vi "Autonomous Turn with Error.vi"(4 "Angle":dbl, 5 "Left Input":dbl, 6 "% Error Margin":dbl, 7 "Right Input":dbl) -> (0 "Left Output":dbl, 1 "Right Output":dbl)   [LabVIEW 2013]
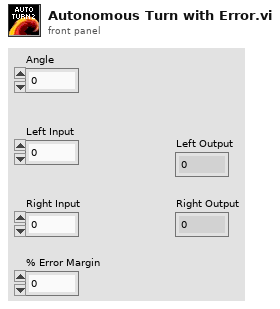
[diagram p1: front panel]
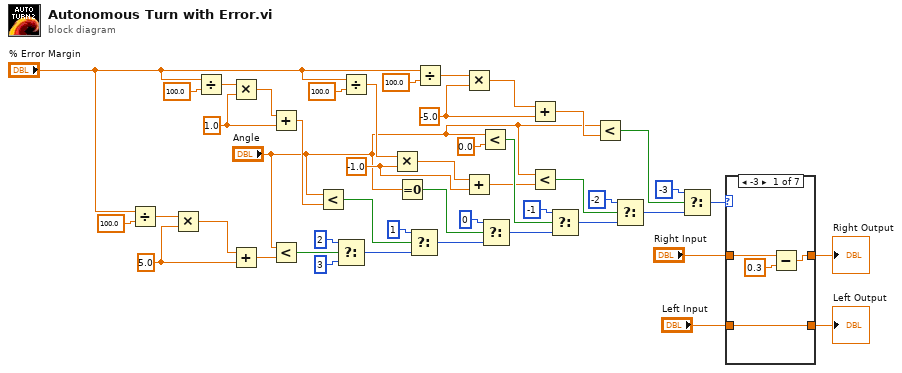
[diagram p0: block diagram]
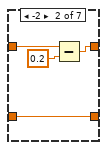
[diagram p2: hidden frame]
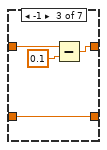
[diagram p3: hidden frame]
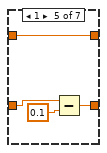
[diagram p5: hidden frame]
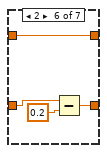
[diagram p6: hidden frame]
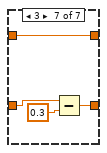
[diagram p7: hidden frame]
diagram:
  w5 = -5.0 ("y")
  w11 = -1.0 ("y")
  w17 = 1.0 ("y")
  w23 = 5.0 ("y")
  n1 = Divide(x="% Error Margin", y=100.0) -> (x/y=w25:dbl)
  n2 = Multiply(x=w25, y=w23) -> (x*y=w24:dbl)
  n3 = Divide(x="% Error Margin", y=100.0) -> (x/y=w19:dbl)
  n4 = Multiply(x=w19, y=w17) -> (x*y=w18:dbl)
  n5 = Add(x=w24, y=w23) -> (x+y=w22:dbl)
  n6 = Add(x=w18, y=w17) -> (x+y=w16:dbl)
  n7 = Less?(x="Angle", y=w22) -> (x < y?=w21:bool)
  n8 = Less?(x="Angle", y=w16) -> (x < y?=w15:bool)
  n9 = Select(t=i8 2, s=w21, f=i8 3) -> (s? t:f=w39:i8)
  n10 = Divide(x="% Error Margin", y=100.0) -> (x/y=w13:dbl)
  n11 = Multiply(x=w13, y=w11) -> (x*y=w12:dbl)
  n12 = Equal To 0?(x="Angle") -> (x = 0?=w35:bool)
  n13 = Select(t=i8 1, s=w15, f=w39) -> (s? t:f=w33:i8)
  n14 = Divide(x="% Error Margin", y=100.0) -> (x/y=w7:dbl)
  n15 = Multiply(x=w7, y=w5) -> (x*y=w6:dbl)
  n16 = Add(x=w12, y=w11) -> (x+y=w10:dbl)
  n17 = Less?(x="Angle", y=0.0) -> (x < y?=w45:bool)
  n18 = Select(t=i8 0, s=w35, f=w33) -> (s? t:f=w32:i8)
  n19 = Add(x=w6, y=w5) -> (x+y=w4:dbl)
  n20 = Less?(x="Angle", y=w10) -> (x < y?=w9:bool)
  n21 = Select(t=i8 -1, s=w45, f=w32) -> (s? t:f=w43:i8)
  n22 = Less?(x="Angle", y=w4) -> (x < y?=w2:bool)
  n23 = Select(t=i8 -2, s=w9, f=w43) -> (s? t:f=w44:i8)
  n24 = Select(t=i8 -3, s=w2, f=w44) -> (s? t:f=w31:i8)
  n25 = case shown="-3" w31 {
    tunnel: "Right Input" -> [w50 w53 w57 w60 w63 w65 w69]
    tunnel: [w48 w52 w56 w60 w63 w65 w69] -> w29
    tunnel: "Left Input" -> [w47 w54 w58 w59 w62 w68 w72]
    tunnel: [w47 w54 w58 w59 w61 w66 w70] -> w27
    frame -3 {
      n26 = Subtract(x=w50, y=0.3) -> (x-y=w48:dbl)
    }
    frame -2 {
      n27 = Subtract(x=w53, y=0.2) -> (x-y=w52:dbl)
    }
    frame -1 {
      n28 = Subtract(x=w57, y=0.1) -> (x-y=w56:dbl)
    }
    frame 0, Default {
    }
    frame 1 {
      n29 = Subtract(x=w62, y=0.1) -> (x-y=w61:dbl)
    }
    frame 2 {
      n30 = Subtract(x=w68, y=0.2) -> (x-y=w66:dbl)
    }
    frame 3 {
      n31 = Subtract(x=w72, y=0.3) -> (x-y=w70:dbl)
    }
  }
  "Left Output" <- w27
  "Right Output" <- w29
